vi "Register Card.vi"(8 "error in (no error)":errorcluster caption="错误输入（无错误）", 10 "card_num":u16, 11 "CardType":u16) -> (0 "error out":errorcluster caption="错误输出", 3 "function return":i16)   [LabVIEW 2017, in "Adlink IO.lvlib"]
doc: "I16 __stdcall Register_Card(U16 CardType, U16 card_num);"
uses:
  Adlink IO.lvlib
  PCI-Dask.dll
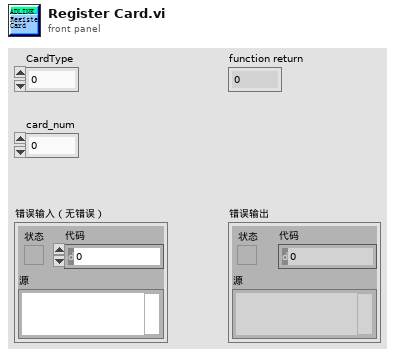
[diagram p1: front panel]
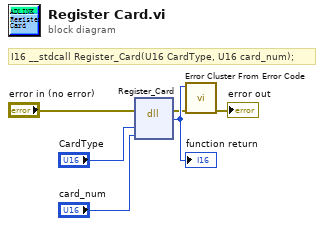
[diagram p0: block diagram]
diagram:
  # "I16 __stdcall Register_Card(U16 CardType, U16 card_num);"
  n1 = dll-call lib="D:/Program/Dyson X692 UI Provison Tester V1.0.0/HardWare/ADLINK/IO/Adlink IO/PCI-Dask.*" fn="Register_Card"(error in="error in (no error)", "CardType"="CardType", "card_num"="card_num") -> (error out=w2:errorcluster, w6:i16)  [unwired: 4 in, 1 out]
  "function return" <- w6
  n2 = call <vilib>:"Error Cluster From Error Code.vi"("error in (no error)"=w2, "error code (0)"=w6) -> ("error out"=→"error out":errorcluster)  [unwired: 7 in]
